vi "DiffDriveVoltageConstraint_getMaxVelocity.vi"(8 "Velocity":dbl, 9 "Curvature":dbl, 10 "statePose":T4={"TRANSLATION"={"X"=0.0, "Y"=0.0}, "ROTATION"={"VALUE"=0.0, "COS"=1.0, "SIN"=0.0}} {"ROTATION"."SIN" format="%13.4f"; "ROTATION"."COS" format="%13.4f"; "ROTATION"."VALUE" format="%13.4f"; "TRANSLATION"."Y" format="%14.3f"; "TRANSLATION"."X" format="%14.3f"}, 11 "DIFF_DRIVE_VOLTAGE_CONSTRAINT":T1 {"SIMPLE_MOTOR_FF"."KnInv" format="%13.4f"; "SIMPLE_MOTOR_FF"."Ka" format="%13.4f"; "SIMPLE_MOTOR_FF"."Kv" format="%13.4f"; "SIMPLE_MOTOR_FF"."Ks" format="%13.4f"; "DIFF_DRIVE_KINEMATICS"."TrackWidth_Meters" format="%20.4f"; "Max Voltage" format="%20.4f"}) -> (3 "absMaxVelocity":dbl)   [LabVIEW 2019, in "Trajectory_Library.lvlib"]
doc: "Return the maximum allowed velocity given the provided conditions.\n\n\nParameters:\n - DiffDriveVoltageConstraint - Constraint data structure\n - statePose - current traj state Pose\n - curvature - current traj curvature\n - maxVelocity - current traj max velocity\n\nReturns\n - maxVelocity - Maximum allowed velocity."
uses:
  Trajectory_Library.lvlib
  TypeDef/TRANSLATION2D.ctl
  TypeDef/ROTATION2D.ctl
  TypeDef/POSE2D.ctl
  TypeDef/DIFF_DRIVE_KINEMATICS.ctl
  TypeDef/SIMPLE_MOTOR_FF.ctl
  TypeDef/TRAJ_CONSTRAINT_DIIF_DRIVE_VOLTAGE.ctl
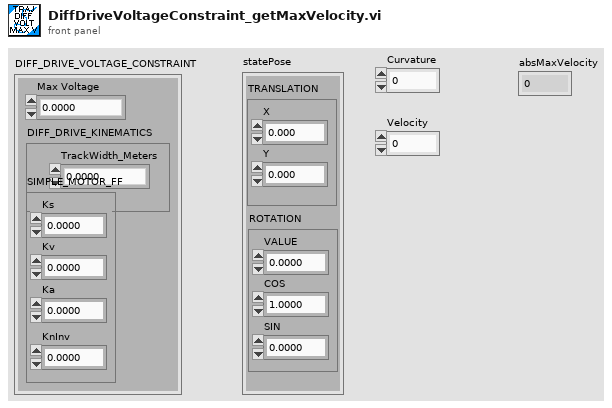
[diagram p1: front panel]
types:
  T1 = typedef "Trajectory_Library.lvlib/TRAJ_CONSTRAINT_DIIF_DRIVE_VOLTAGE.ctl" = cluster{"Max Voltage":dbl, "DIFF_DRIVE_KINEMATICS":T2, "SIMPLE_MOTOR_FF":T3}
  T2 = typedef "Trajectory_Library.lvlib/DIFF_DRIVE_KINEMATICS.ctl" = cluster{"TrackWidth_Meters":dbl}
  T3 = typedef "Trajectory_Library.lvlib/SIMPLE_MOTOR_FF.ctl" = cluster{"Ks":dbl, "Kv":dbl, "Ka":dbl, "KnInv":dbl}
  T4 = typedef "Trajectory_Library.lvlib/POSE2D.ctl" = cluster{"TRANSLATION":T5, "ROTATION":T6}
  T5 = typedef "Trajectory_Library.lvlib/TRANSLATION2D.ctl" = cluster{"X":dbl, "Y":dbl}
  T6 = typedef "Trajectory_Library.lvlib/ROTATION2D.ctl" = cluster{"VALUE":dbl, "COS":dbl, "SIN":dbl}
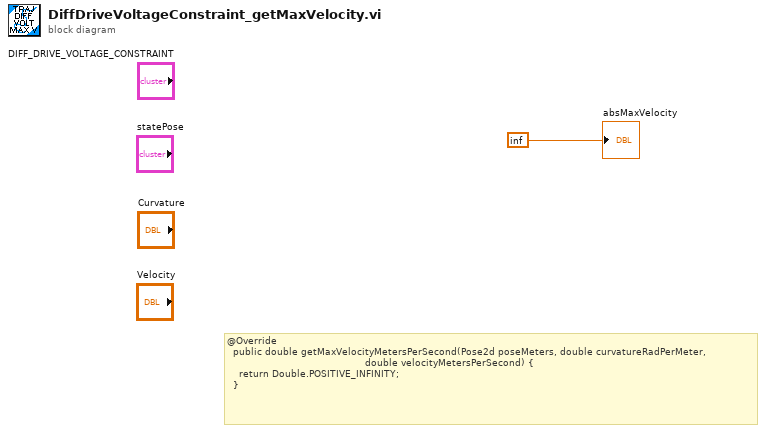
[diagram p0: block diagram]
diagram:
  # "@Override\n  public double getMaxVelocityMetersPerSecond(Pose2d poseMeters, double curvatureRadPerMeter,\n                                              double velocityMetersPerSecond) {\n    return Double.POSITIVE_INFINITY;\n  }"
  "absMaxVelocity" <- inf
